vi "Examen.vi"() -> ()   [LabVIEW 2020]
uses:
  <vilib>/numeric/Random Number (Range) U64.vi
  <vilib>/numeric/sub_Random U32.vi
panel:
  out "EMA":dbl[](array[numeric])
  out "Contador":dbl
  out "Waveform Chart":dynamicdata(graph)
  out "Valor":dbl
  in  "stop":bool
  out "Dentro del rango":bool
  out "Histeresis":bool
  in  "Minimo":dbl
  in  "Maximo":dbl
  out "Numero":u64
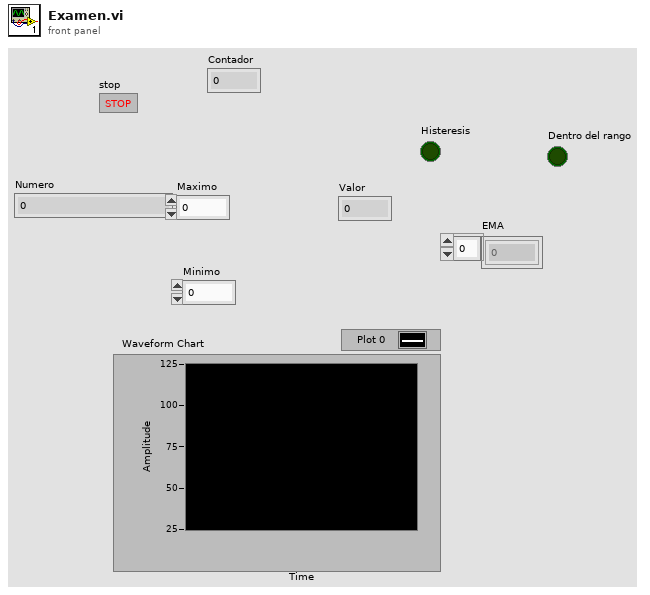
[diagram p1: front panel]
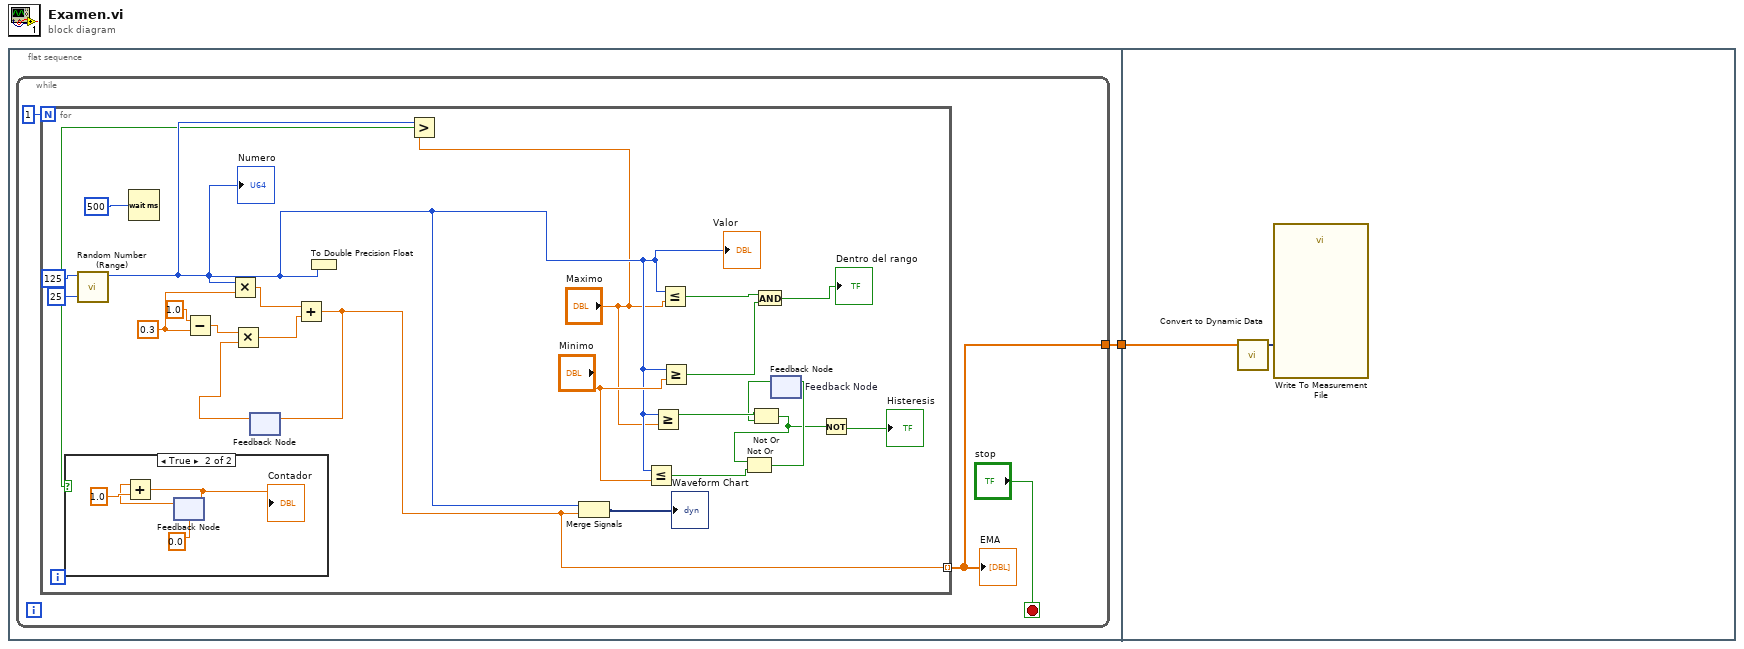
[diagram p0: block diagram]
diagram:
  n1 = flat-sequence {
    tunnel: [w2] -> w1
    tunnel: w1 -> [w35]
    frame #0 {
      n2 = while {
        tunnel: [w4] -> w2
        stop <- "stop" stop-if-true
        n3 = for {
          N: 1 -> [_]
          tunnel: [w6] -> w4 mode=indexing
          w22 = 0.3 ("y")
          n4 = call-poly <vilib>:"Random Number (Range).vi"("lower bound (0)"=u64 25, "upper bound (100)"=u64 125) -> ("number"=w9:u64)  [unwired: 9 in]
          "Numero" <- w9
          "Valor" <- w9
          n5 = Wait (ms)(milliseconds to wait=u32 500 ("millisecond timer value")) -> ()  [unwired: 1 out]
          n6 = Subtract(x=1.0, y=w22) -> (x-y=w26:dbl)
          n7 = Multiply(x=w9, y=w22) -> (x*y=w23:dbl)
          n8 = feedback #1() -> (w10:dbl)  [unwired: 1 in]
          n9 = Multiply(x=w26, y=w10) -> (x*y=w24:dbl)
          n10 = Add(x=w23, y=w24) -> (x+y=w6:dbl)
          n11 = feedback-in #1(w6) -> ()
          n12 = To Double Precision Float(number=w9) -> ()  [unwired: 1 out]
          n13 = Greater?(x=w9, y="Maximo") -> (0:w7:bool)
          n14 = case shown="True" w7 {
            frame False {
            }
            frame True {
              n15 = feedback #2(0.0) -> (w31:dbl)
              n16 = Add(x=w31, y=1.0) -> (x+y=w30:dbl)
              "Contador" <- w30
              n17 = feedback-in #2(w30) -> ()
            }
          }
          n18 = Merge Signals "Merge Signals"(w9, w6) -> (→"Waveform Chart":dynamicdata)
          n19 = Less Or Equal?(x=w9, y="Minimo") -> (x <= y?=w14:bool)
          n20 = Greater Or Equal?(x=w9, y="Maximo") -> (x >= y?=w15:bool)
          n21 = Less Or Equal?(x=w9, y="Maximo") -> (x <= y?=w20:bool)
          n22 = Greater Or Equal?(x=w9, y="Minimo") -> (x >= y?=w19:bool)
          n23 = And(x=w20, y=w19) -> (x .and. y?=→"Dentro del rango":bool)
          n24 = feedback #3 "Feedback Node"() -> (w13:bool)  [unwired: 1 in]
          n25 = Not Or(1:w13, 2:w15) -> (0:w12:bool)
          n26 = Not Or(1:w14, 2:w12) -> (0:w17:bool)
          n27 = feedback-in #3(w17) -> ()
          n28 = Not(x=w12) -> (.not. x?=→"Histeresis":bool)
        }
        "EMA" <- w4
      }
    }
    frame #1 {
      n29 = call "Convert to Dynamic Data"("Array"=w35) -> ("Dynamic Data Type"=w34:dynamicdata)  [unwired: 3 in]
      n30 = call "Write To Measurement File"("Signals"=w34) -> ()  [unwired: 16 in, 3 out]
    }
  }
